vi "Solar Panel.vi"(11 "Time in Hours":u32) -> (3 "String":string)   [LabVIEW 2021]
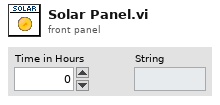
[diagram p1: front panel]
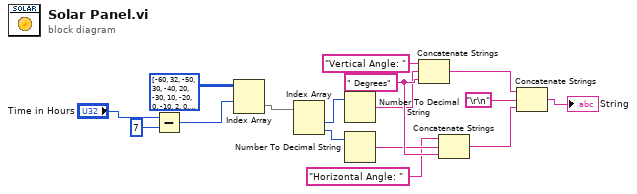
[diagram p0: block diagram]
diagram:
  w11 = " Degrees" ("string")
  n1 = Subtract(x="Time in Hours", y=u32 7) -> (x-y=w3:u32)
  n2 = Index Array(array=i32[][] [[-60, 32], [-50, 30], [-40, 20], [-30, 10], [-20, 0], [-10, 2], [0, 5], [10, 9], [20, 11], [30, 13], [40, 15], [50, 18], [0, 0]] ("initialized array"), index (row)=w3) -> (element=w4:i32[])  [unwired: 1 in]
  n3 = Index Array(array=w4) -> (element #1=w6:i32, element #2=w7:i32)  [unwired: 2 in]
  n4 = Number To Decimal String(number=w6) -> (decimal integer string=w8:string)  [unwired: 1 in]
  n5 = Number To Decimal String(number=w7) -> (decimal integer string=w10:string)  [unwired: 1 in]
  n6 = Concatenate Strings("Vertical Angle: " ("string"), w8, w11) -> (w12:string)
  n7 = Concatenate Strings("Horizontal Angle: " ("string"), w10, w11) -> (w14:string)
  n8 = Concatenate Strings(w12, "\r\n", w14) -> (→"String":string)
